vi "DriveControlLoop.vi"() -> ()   [LabVIEW 2018]
uses:
  <vilib>/Rock Robotics/WPI/ThirdParty/Phoenix-LabVIEW/Motor Controller/Controls/CTRE_Phoenix_MotorControl_ControlMode.ctl
  Infrastructure/RobotMap.vi
  <vilib>/Rock Robotics/Network Tables/NT Write Number.vi
  Robot Global Data.vi
  <vilib>/Rock Robotics/WPI/ThirdParty/Phoenix-LabVIEW/Motor Controller/Get/CTRE_Phoenix_MotorController_GetSelectedSensorData.vi
  <vilib>/Rock Robotics/WPI/ThirdParty/Phoenix-LabVIEW/Motor Controller/Get/CTRE_Phoenix_MotorController_GetOutputCurrent_Enhanced.vi
  <vilib>/Rock Robotics/Network Tables/NT Write Boolean.vi
panel:
  out "MM on last step":bool
  out "Index of Current Auton Step":dbl
  out "Hab2toHab1Step":enum16{"Go Forward", "Go Backward", "Set Home"}(ring)
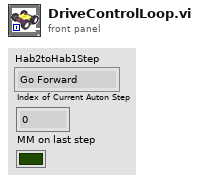
[diagram p1: front panel]
types:
  T1 = typedef "WPI_MotorControlDeviceRef.ctl" = cluster{"DeviceStatus":errorcluster, "Type":T2, "PWM":cluster{"PWM Channel":T3, "DeadBand":T4}, "CAN":cluster{"Device Number":u8, "SetOutput VI Ref":variant, "GetOutput VI Ref":variant, "Enable VI Ref":variant, "Disable VI Ref":variant, "Data":variant}, "Invert":bool, "DIO PWM":cluster{"PWM \"Enable\" Channel":T3, "DIOChannel":T5, "PWM Rate":dbl}}
  T2 = typedef "WPI_MotorControlType.ctl" = enum16{"PWM", "CAN", "DIO PWM"}
  T3 = typedef "FPGA_DIOPWMChannel.ctl" = enum8{"PWM 0", "PWM 1", "PWM 2", "PWM 3", "PWM 4", "PWM 5", "PWM 6", "PWM 7", "PWM 8", "PWM 9", "PWM MXP 0", "PWM MXP 1", "PWM MXP 2", "PWM MXP 3", "PWM MXP 4", "PWM MXP 5", "PWM MXP 6", "PWM MXP 7", "PWM MXP 8", "PWM MXP 9", "Invalid"}
  T4 = typedef "WPI_PWMDeadband.ctl" = cluster{"Name":string, "maxPositivePwm":i32, "minPositivePwm":i32, "centerPwm":i32, "maxNegativePwm":i32, "minNegativePwm":i32, "angularRange":u16}
  T5 = typedef "FPGA_DIOChannel.ctl" = enum8{"DIO 0", "DIO 1", "DIO 2", "DIO 3", "DIO 4", "DIO 5", "DIO 6", "DIO 7", "DIO 8", "DIO 9", "DIO MXP 0", "DIO MXP 1", "DIO MXP 2", "DIO MXP 3", "DIO MXP 4", "DIO MXP 5", "DIO MXP 6", "DIO MXP 7", "DIO MXP 8", "DIO MXP 9", "DIO MXP 10", "DIO MXP 11", "DIO MXP 12", "DIO MXP 13", "DIO MXP 14", "DIO MXP 15", "SPI Port CS1", "SPI Port CS2", "SPI Port CS3", "SPI Port MISO", "SPI Port MOSI", "Invalid"}
  T6 = typedef "WPI_GyroDevRef.ctl" = cluster{"DevStatus":errorcluster, "Analog Channel":T7, "Gain (VoltsPerDegree/Second)":dbl, "Gyro Type":enum16{"Analog", "XRS450"}, "Handle":i32, "SPI Bus":T8, "Device Found":bool, "Sample Rate":dbl, "Calibrate On Open":bool, "Offset":dbl}
  T7 = typedef "FPGA_AIChannel.ctl" = enum8{"AI 0", "AI 1", "AI 2", "AI 3", "AI MXP 0", "AI MXP 1", "AI MXP 2", "AI MXP 3", "Invalid"}
  T8 = typedef "spi_bus.ctl" = enum16{"SPI On-Board, CS0", "SPI On-Board, CS1", "SPI On-Board, CS2", "SPI On-Board, CS3", "SPI MXP", "Invalid"}
  T9 = cluster{"Position (Raw Sensor Units)":i32, "Velocity (Raw Sensor Units per 100 ms)":i32}
  T10 = typedef "Drive mode.ctl" = enum16{"HAB2toHAB1", "Driver Operated", "Drive Autonomously", "Disabled"}
  T11 = typedef "CTRE_Phoenix_MotorControl_ControlMode.ctl" = u16
  T12 = cluster{"Left Motor Value":dbl, "Right Motor Value":dbl}
  T13 = typedef "Drive Motion Magic Setpoints.ctl" = cluster{"Increase in Left":dbl, "Increase in Right":dbl}[]
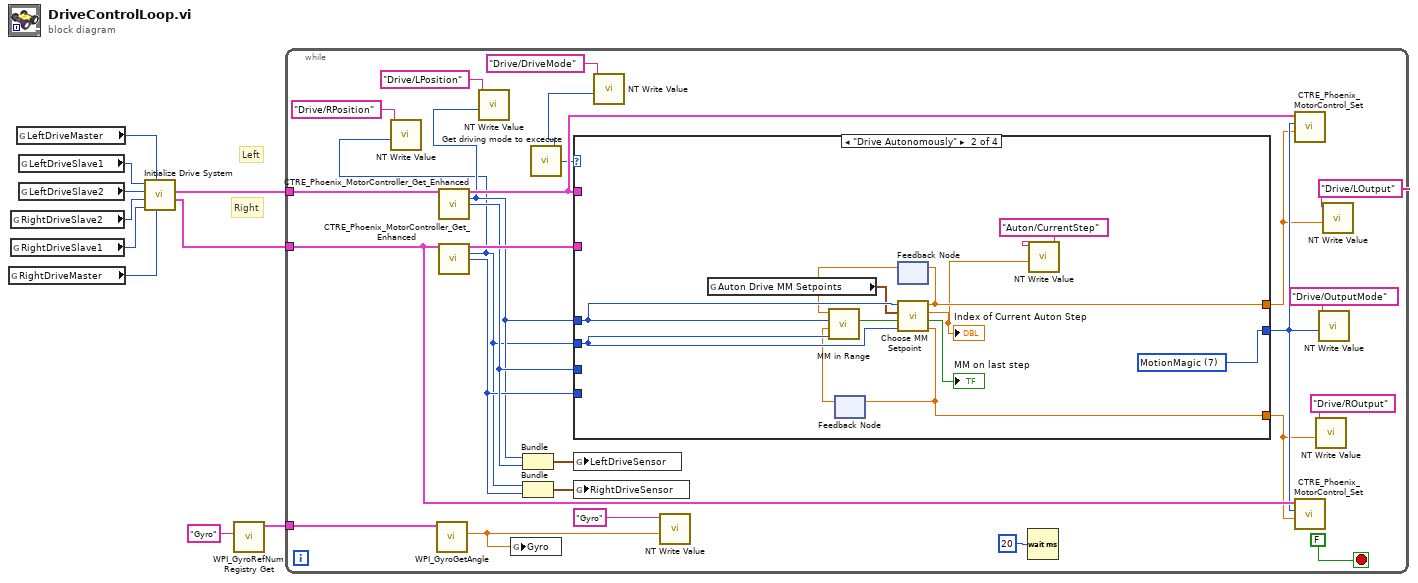
[diagram p0: block diagram]
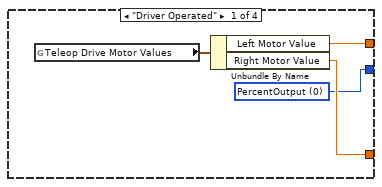
[diagram p2: hidden frame]
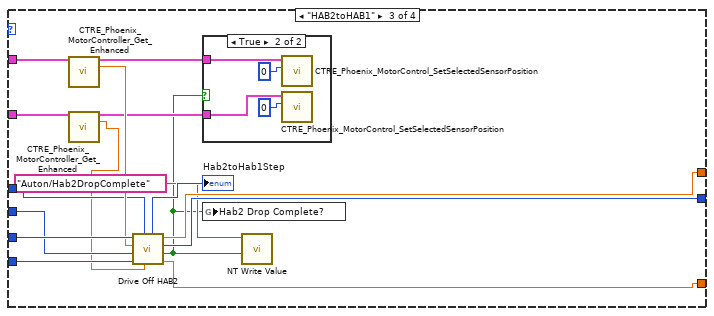
[diagram p3: hidden frame]
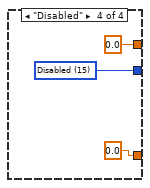
[diagram p5: hidden frame]
diagram:
  # "Right"
  # "Left"
  n1 = global read "RobotMap.vi" "RightDriveMaster"() -> (w8:u8)
  n2 = global read "RobotMap.vi" "RightDriveSlave2"() -> (w10:u8)
  n3 = global read "RobotMap.vi" "RightDriveSlave1"() -> (w9:u8)
  n4 = global read "RobotMap.vi" "LeftDriveMaster"() -> (w5:u8)
  n5 = global read "RobotMap.vi" "LeftDriveSlave1"() -> (w6:u8)
  n6 = global read "RobotMap.vi" "LeftDriveSlave2"() -> (w7:u8)
  n7 = call "Initialize Drive System.vi"("RightDriveMaster"=w8, "LeftDriveMaster"=w5, "RightDriveSlave1"=w9, "RightDriveSlave2"=w10, "LeftDriveSlave 2"=w7, "LeftDriveSlave1"=w6) -> ("RightDriveMaster"=w3:T1, "LeftDriveMaster"=w4:T1)  [unwired: 4 in]
  n8 = call <vilib>:"WPI_GyroRefNum Registry Get.vi"("refnum name"="Gyro") -> ("GyroDevRef"=w1:T6)  [unwired: 9 in, 1 out]
  n9 = while {
    tunnel: w4 -> [w27]
    tunnel: w3 -> [w26]
    tunnel: w1 -> [w33]
    stop <- FALSE stop-if-true
    n10 = call <vilib>:"WPI_GyroGetAngle.vi"("GyroDevRef"=w33) -> ("Angle"=w24:dbl)  [unwired: 6 in, 4 out]
    n11 = call-poly <vilib>:"CTRE_Phoenix_MotorController_Get_Enhanced.vi"("PhoenixMotorControlDevRef"=w27) -> ("PhoenixMotorControlDevRef"=w31:T1, "Position (Raw Sensor Units)"=w19:i32, "Velocity (Raw Sensor Units per 100 ms)"=w29:i32)  [unwired: 11 in, 1 out]
    n12 = call-poly <vilib>:"CTRE_Phoenix_MotorController_Get_Enhanced.vi"("PhoenixMotorControlDevRef"=w26) -> ("PhoenixMotorControlDevRef"=w32:T1, "Position (Raw Sensor Units)"=w17:i32, "Velocity (Raw Sensor Units per 100 ms)"=w25:i32)  [unwired: 11 in, 1 out]
    n13 = call-poly <vilib>:"NT Write Value.vi"("Numeric"=w17, "Name"="Drive/RPosition") -> ()  [unwired: 9 in, 1 out]
    n14 = call-poly <vilib>:"NT Write Value.vi"("Numeric"=w19, "Name"="Drive/LPosition") -> ()  [unwired: 9 in, 1 out]
    n15 = global write "Robot Global Data.vi" "Gyro"(w24) -> ()
    n16 = Bundle("Position (Raw Sensor Units)"=w19, "Velocity (Raw Sensor Units per 100 ms)"=w29) -> (w30:T9)  [unwired: 1 in]
    n17 = Bundle("Position (Raw Sensor Units)"=w17, "Velocity (Raw Sensor Units per 100 ms)"=w25) -> (w28:T9)  [unwired: 1 in]
    n18 = call "Get driving mode to excecute.vi"() -> ("Drive Mode"=w21:T10)  [unwired: 1 in]
    n19 = case shown="\"Drive Autonomously\"" w21 {
      tunnel: w19 -> [_ w50 w63 _]
      tunnel: [w38 w44 w58 0.0 ("Left Motor Value")] -> w13
      tunnel: [w36 w51 w57 w74] -> w15
      tunnel: w17 -> [_ w49 w62 _]
      tunnel: [w37 w46 w56 0.0 ("Right Motor Value")] -> w11
      tunnel: w29 -> [_ _ w65 _]
      tunnel: w25 -> [_ _ w61 _]
      tunnel: w31 -> [_ _ w67 _]
      tunnel: w32 -> [_ _ w66 _]
      frame "Driver Operated" {
        w36 = T11 0 items=["PercentOutput"=0, "Position"=1, "Velocity"=2, "Current"=3, "Follower"=5, "MotionProfile"=6, "MotionMagic"=7, "MotionProfileArc"=10, "Disabled"=15] ("Control Mode")
        n20 = global read "Robot Global Data.vi" "Teleop Drive Motor Values"() -> (w39:T12)
        n21 = Unbundle By Name(w39) -> ("Left Motor Value"=w38:dbl, "Right Motor Value"=w37:dbl)
      }
      frame "Drive Autonomously" {
        w51 = T11 7 items=["PercentOutput"=0, "Position"=1, "Velocity"=2, "Current"=3, "Follower"=5, "MotionProfile"=6, "MotionMagic"=7, "MotionProfileArc"=10, "Disabled"=15] ("Control Mode")
        n22 = global read "Robot Global Data.vi" "Auton Drive MM Setpoints"() -> (w47:T13)
        n23 = feedback #1() -> (w45:dbl)  [unwired: 1 in]
        n24 = feedback #2() -> (w43:dbl)  [unwired: 1 in]
        n25 = call "MM in Range.vi"("Right Position"=w49, "Right Setpoint"=w45, "Left position"=w50, "Left Setpoint"=w43) -> ("\"Done with step\" enough"=w48:bool)  [unwired: 7 in]
        n26 = call "Choose MM Setpoint.vi"("Right Encoder Pos"=w49, "\"Done with step\" enough"=w48, "Steps"=w47, "Left Encoder Pos"=w50) -> ("Right Motor Setpoint"=w46:dbl, "MM on last step"=→"MM on last step":bool, "Index of Current Step"=w40:dbl, "Left Motor Setpoint"=w44:dbl)  [unwired: 4 in]
        "Index of Current Auton Step" <- w40
        n27 = feedback-in #1(w46) -> ()
        n28 = feedback-in #2(w44) -> ()
        n29 = call-poly <vilib>:"NT Write Value.vi"("Numeric"=w40, "Name"="Auton/CurrentStep") -> ()  [unwired: 9 in, 1 out]
      }
      frame "HAB2toHAB1" {
        n30 = call-poly <vilib>:"CTRE_Phoenix_MotorController_Get_Enhanced.vi"("PhoenixMotorControlDevRef"=w67) -> ("PhoenixMotorControlDevRef"=w55:T1, "Output Current"=w64:dbl)  [unwired: 12 in, 1 out]
        n31 = call-poly <vilib>:"CTRE_Phoenix_MotorController_Get_Enhanced.vi"("PhoenixMotorControlDevRef"=w66) -> ("PhoenixMotorControlDevRef"=w54:T1, "Output Current"=w60:dbl)  [unwired: 12 in, 1 out]
        n32 = call "Drive Off HAB2.vi"("Right Current Drawn"=w60, "Left Position"=w63, "Right Velocity"=w61, "Right Position"=w62, "Left Current Drawn"=w64, "Left Velocity"=w65) -> ("Right Output"=w56:dbl, "Zero Encoders"=w52:bool, "Control Mode"=w57:T11, "Left Output"=w58:dbl, "Step"=→"Hab2toHab1Step":enum16{"Go Forward", "Go Backward", "Set Home"})  [unwired: 1 out]
        n33 = case shown="True" w52 {
          tunnel: w55 -> [_ w69]
          tunnel: w54 -> [_ w68]
          frame False {
          }
          frame True {
            n34 = call <vilib>:"CTRE_Phoenix_MotorControl_SetSelectedSensorPosition.vi"("New Sensor Position"=0, "PhoenixMotorControlDevRef"=w69) -> ()  [unwired: 8 in, 2 out]
            n35 = call <vilib>:"CTRE_Phoenix_MotorControl_SetSelectedSensorPosition.vi"("New Sensor Position"=0, "PhoenixMotorControlDevRef"=w68) -> ()  [unwired: 8 in, 2 out]
          }
        }
        n36 = global write "Robot Global Data.vi" "Hab2 Drop Complete?"(w52) -> ()
        n37 = call-poly <vilib>:"NT Write Value.vi"("Boolean"=w52, "Name"="Auton/Hab2DropComplete") -> ()  [unwired: 9 in, 1 out]
      }
      frame "Disabled" {
        w74 = T11 15 items=["PercentOutput"=0, "Position"=1, "Velocity"=2, "Current"=3, "Follower"=5, "MotionProfile"=6, "MotionMagic"=7, "MotionProfileArc"=10, "Disabled"=15] ("Control Mode")
      }
    }
    n38 = global write "Robot Global Data.vi" "LeftDriveSensor"(w30) -> ()
    n39 = global write "Robot Global Data.vi" "RightDriveSensor"(w28) -> ()
    n40 = call-poly <vilib>:"NT Write Value.vi"("Numeric"=w21, "Name"="Drive/DriveMode") -> ()  [unwired: 9 in, 1 out]
    n41 = call-poly <vilib>:"NT Write Value.vi"("Numeric"=w24, "Name"="Gyro") -> ()  [unwired: 9 in, 1 out]
    n42 = Wait (ms)(milliseconds to wait=u32 20) -> ()  [unwired: 1 out]
    n43 = call <vilib>:"CTRE_Phoenix_MotorControl_Set.vi"("Output"=w13, "Control Mode"=w15, "PhoenixMotorControlDevRef"=w31) -> ()  [unwired: 7 in, 2 out]
    n44 = call <vilib>:"CTRE_Phoenix_MotorControl_Set.vi"("Output"=w11, "Control Mode"=w15, "PhoenixMotorControlDevRef"=w26) -> ()  [unwired: 7 in, 2 out]
    n45 = call-poly <vilib>:"NT Write Value.vi"("Numeric"=w11, "Name"="Drive/ROutput") -> ()  [unwired: 9 in, 1 out]
    n46 = call-poly <vilib>:"NT Write Value.vi"("Numeric"=w15, "Name"="Drive/OutputMode") -> ()  [unwired: 9 in, 1 out]
    n47 = call-poly <vilib>:"NT Write Value.vi"("Numeric"=w13, "Name"="Drive/LOutput") -> ()  [unwired: 9 in, 1 out]
  }
